vi "Dialog Window flow test.vi"(6 "Error In":errorcluster) -> (0 "Error Out":errorcluster)   [LabVIEW 2014]
panel:
  out "Üzenet":string
  in  "OK":bool
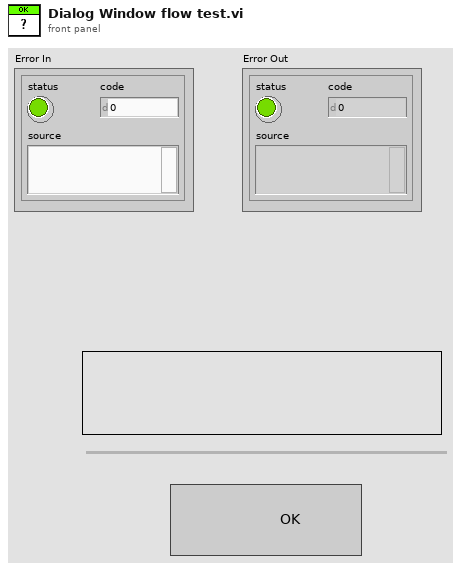
[diagram p1: front panel]
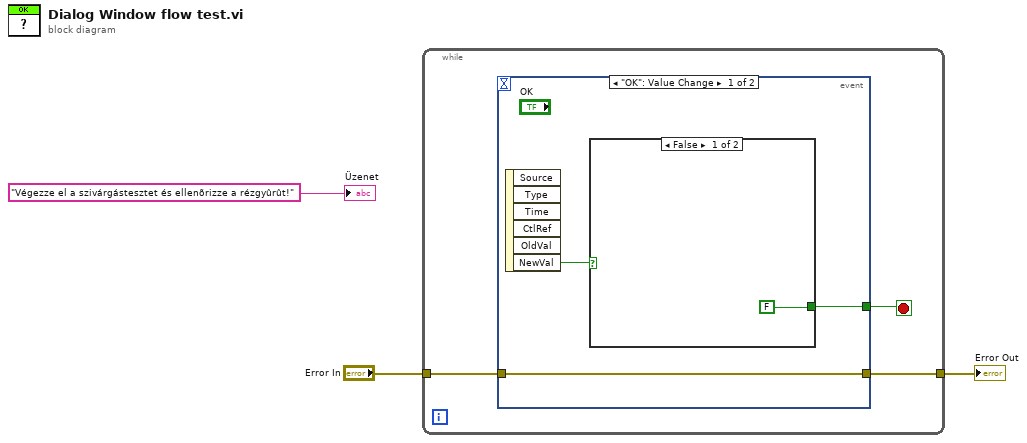
[diagram p0: block diagram]
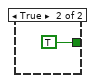
[diagram p2: hidden frame]
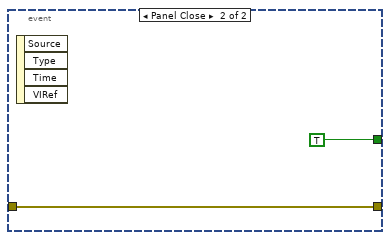
[diagram p3: hidden frame]
diagram:
  n1 = while {
    tunnel: "Error In" -> [w6]
    tunnel: [w5] -> w3
    stop <- w4 stop-if-true
    n2 = event shown="[0] \"OK\": Value Change" {
      selector: _ -> [_ _]
      dyn-events: _ -> [_ _]
      timeout: _ -> [_ _]
      tunnel: [w9 w13] -> w5
      tunnel: w6 -> [w9 w13]
      tunnel: [w7 TRUE] -> w4
      event "OK": Value Change {
        n3 = event-data() -> ("NewVal"=w8:bool)  [unwired: 1 in, 5 out]
        n4 = case shown="False" w8 {
          tunnel: [FALSE TRUE] -> w7
          frame False {
          }
          frame True {
          }
        }
      }
      event Panel Close {
        n5 = event-data() -> ()  [unwired: 1 in, 4 out]
      }
    }
  }
  "Error Out" <- w3
  "Üzenet" <- "Végezze el a szivárgástesztet és ellenõrizze a rézgyûrût!" ("Üzenet")
